vi "Scaled Picture Co-ordinates to Image Co-ordinates.vi"(1 "Image Draw Offset":T4, 2 "Picture Control Coords":T2, 4 "Border Thickness (Default: 2,3)":T1={"Width"=1, "Height"=3}, 5 "Zoom Factor Set":dbl) -> (7 "Image Point":T3)   [LabVIEW 2020, in "image.lvlib"]
doc: "Convert from a LabVIEW Picture Co-ordinate with a Zoom Factor and Drawing Offset to Image Co-ordinates."
uses:
  Image Draw Offset.ctl
  common/Image Point (Float).ctl
  <vilib>/Utility/miscctls.llb/LVPoint32TypeDef.ctl
  common/Image Size (Integer).ctl
  image.lvlib
  common/common.lvlib
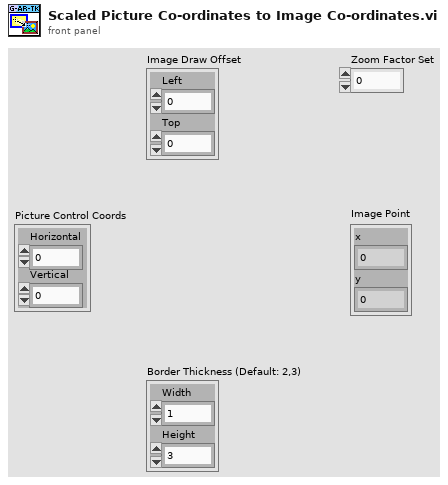
[diagram p1: front panel]
types:
  T1 = typedef "common.lvlib/Image Size (Integer).ctl" = cluster{"Width":u16, "Height":u16}
  T2 = typedef "LVPoint32TypeDef.ctl" = cluster{"Horizontal":i32, "Vertical":i32}
  T3 = typedef "common.lvlib/Image Point (Float).ctl" = cluster{"x":dbl, "y":dbl}
  T4 = typedef "image.lvlib/Image Draw Offset.ctl" = cluster{"Left":i16, "Top":i16}
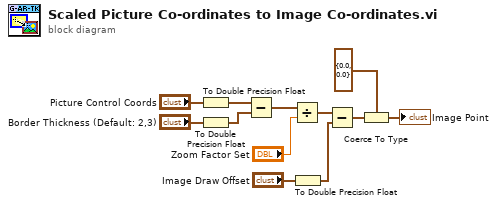
[diagram p0: block diagram]
diagram:
  n1 = To Double Precision Float(number="Picture Control Coords") -> (double precision float=w7:cluster{"Horizontal":dbl, "Vertical":dbl})
  n2 = To Double Precision Float(number="Border Thickness (Default: 2,3)") -> (double precision float=w1:cluster{"Width":dbl, "Height":dbl})
  n3 = Subtract(x=w7, y=w1) -> (x-y=w2:cluster{dbl, dbl})
  n4 = Divide(x=w2, y="Zoom Factor Set") -> (x/y=w10:cluster{dbl, dbl})
  n5 = To Double Precision Float(number="Image Draw Offset") -> (double precision float=w6:cluster{"Left":dbl, "Top":dbl})
  n6 = Subtract(x=w10, y=w6) -> (x-y=w9:cluster{dbl, dbl})
  n7 = Coerce To Type(0:w9, 1:T3 {"x"=0.0, "y"=0.0} ("Image Point")) -> (2:→"Image Point":T3)
